vi "C867_Stop.vi"(8 "error in":errorcluster caption="entrée d'erreur") -> (0 "error out":errorcluster caption="sortie d'erreur")   [LabVIEW 2026]
panel:
  out "return code":i32 caption="code de retour"
  out "standard error":string caption="erreur standard"
  out "standard output":string caption="sortie standard"
  out "chaîne concaténée":string
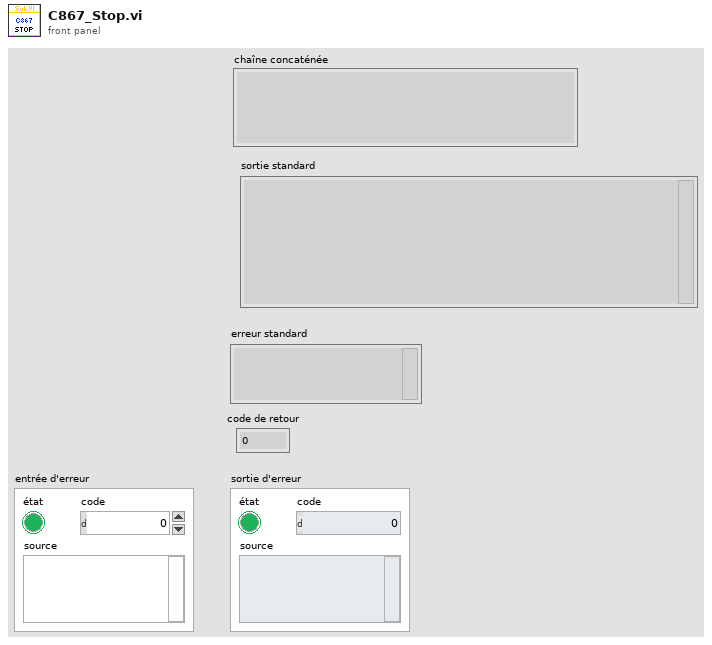
[diagram p1: front panel]
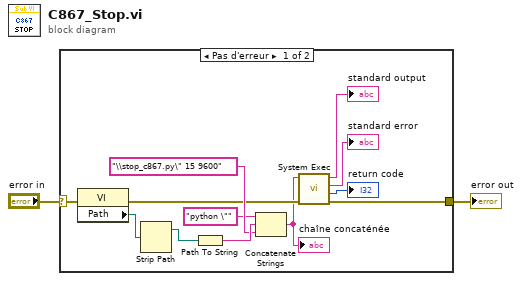
[diagram p0: block diagram]
diagram:
  n1 = case shown="Pas d'erreur" "error in" {
    selector: "error in" -> [w10 w15]
    tunnel: [w8 w15] -> w1
    frame No Error {
      n2 = property class="VI"(error in=w10) -> (error out=w9:errorcluster, "Path"=w13:path)  [unwired: 1 in, 1 out]
      n3 = Strip Path(path=w13) -> (stripped path=w14:path)  [unwired: 1 out]
      n4 = Path To String(path=w14) -> (string=w12:string)
      n5 = Concatenate Strings("python \"" ("string"), w12, "\\stop_c867.py\" 15 9600" ("string")) -> (w7:string)
      "chaîne concaténée" <- w7
      n6 = call <vilib>:"System Exec.vi"("error in (no error)"=w9, "command line"=w7) -> ("error out"=w8:errorcluster, "return code"=→"return code":i32, "standard error"=→"standard error":string, "standard output"=→"standard output":string)  [unwired: 6 in]
    }
    frame Error {
    }
  }
  "error out" <- w1
